vi "Write system error.vi"(8 "error in (no error)":errorcluster, 11 "Channel in":refnum<class "SPARC4_Channel.lvclass">) -> (0 "error out":errorcluster, 3 "Channel out":refnum<class "SPARC4_Channel.lvclass">)   [LabVIEW 2018, in "SPARC4_Channel.lvclass"]
uses:
  SPARC4_Channel.lvclass
  SPARC4_Channel.lvclass/SPARC4_Channel.ctl
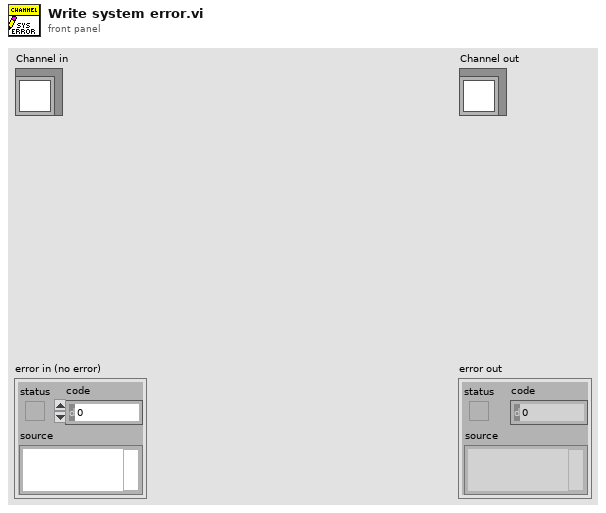
[diagram p1: front panel]
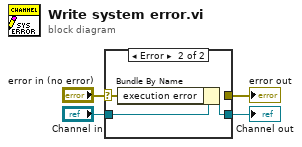
[diagram p0: block diagram]
diagram:
  n1 = case shown="Error" "error in (no error)" {
    selector: "error in (no error)" -> [w6 w7]
    tunnel: [w6 _] -> w3
    tunnel: [w5 w8] -> w1
    tunnel: "Channel in" -> [w5 w9]
    frame No Error {
    }
    frame Error {
      n2 = Bundle By Name(cluster=w9, "execution error"=w7) -> (w8:refnum<class "SPARC4_Channel.lvclass">)
    }
  }
  "error out" <- w3
  "Channel out" <- w1
